vi "Initialize.vi"(8 "Error In":errorcluster, 11 "Initialization Data":variant) -> (0 "Error Out":errorcluster)   [LabVIEW 2012, in "CS++MessageLogger.lvlib"]
doc: "Initialize the central message logger."
uses:
  CS++MessageLogger.lvlib
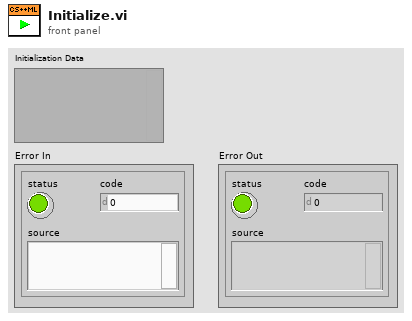
[diagram p1: front panel]
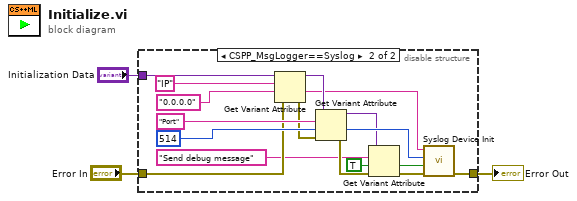
[diagram p0: block diagram]
diagram:
  n1 = disable-structure shown="CSPP_MsgLogger==Syslog" {
    disable-tunnel: "Error In" -> [w4 w9]
    disable-tunnel: [w4 w21] -> w2
    disable-tunnel: "Initialization Data" -> [_ w20]
    frame condition #0 {
    }
    frame condition #1 (active) {
      n2 = Get Variant Attribute(Variant=w20, name="IP", default value (empty Variant)="0.0.0.0" ("name"), error in=w9) -> (duplicate Variant=w16:variant, value=w13:string, error out=w14:errorcluster)  [unwired: 1 out]
      n3 = Get Variant Attribute(Variant=w16, name="Port", default value (empty Variant)=u16 514 ("Collector Port (514)"), error in=w14) -> (duplicate Variant=w11:variant, value=w12:u16, error out=w10:errorcluster)  [unwired: 1 out]
      n4 = Get Variant Attribute(Variant=w11, name="Send debug message", default value (empty Variant)=TRUE, error in=w10) -> (value=w5:bool, error out=w8:errorcluster)  [unwired: 2 out]
      n5 = call <userlib>:"Syslog Device Init.vi"("error in (no error)"=w8, "Send debug message (T)"=w5, "Collector Port (514)"=w12, "Syslog Collector IP Address"=w13) -> ("error out"=w21:errorcluster)  [unwired: 7 in]
    }
  }
  "Error Out" <- w2
